vi "Initialise.vi"(8 "error in (no error)":errorcluster, 11 "JsonEvents in":refnum<class "JsonEvents.lvclass">) -> (0 "error out":errorcluster, 3 "JsonEvents out":refnum<class "JsonEvents.lvclass">)   [LabVIEW 2020, in "wamplv.lvlib" / "JsonEvents.lvclass"]
uses:
  JsonEvents.lvclass
  WAMP Client/Private/TypeDef/EVENT payload (JSON).ctl
  WAMP Client/API/TypeDefs/INVOCATION payload.ctl
  Invocation Request ID/Invocation Request ID.lvclass
  WAMP Client/API/TypeDefs/RESULT payload (JSON).ctl
  WAMP Client/API/TypeDefs/Error or abort detail (JSON).ctl
  JsonEvents.lvclass/JsonEvents.ctl
  EventsParent/Events.lvclass
  wamplv.lvlib
  WAMP Client/WAMP Client.lvclass
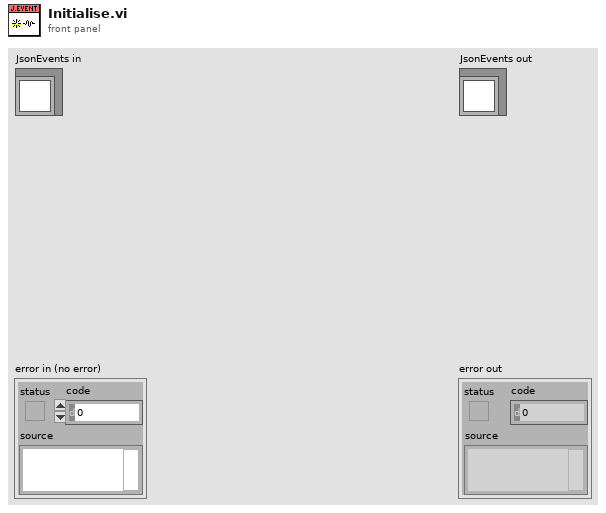
[diagram p1: front panel]
types:
  T1 = typedef "wamplv.lvlib/EVENT payload (JSON).ctl" = cluster{"Publication ID":u64, "Topic":string, "Arguments Payload":string, "ArgumentKw Payload":string, "Details":string}
  T2 = typedef "wamplv.lvlib/WAMP Client.lvclass/INVOCATION payload.ctl" = cluster{"Arguments":string, "ArgumentKw":string, "Procedure URI":string, "Details":string, "Registration ID":u64, "Invocation Request ID":refnum<class "Invocation Request ID.lvclass">}
  T3 = typedef "wamplv.lvlib/WAMP Client.lvclass/RESULT payload (JSON).ctl" = cluster{"Topic":string, "Arguments Payload":string, "ArgumentKw Payload":string, "Details":string, "Error/Abort details (JSON)":T4}
  T4 = typedef "wamplv.lvlib/Error or abort detail (JSON).ctl" = cluster{"Error URI":string, "Error Arguments":string, "Error ArgumentKw":string, "Error Details":string}
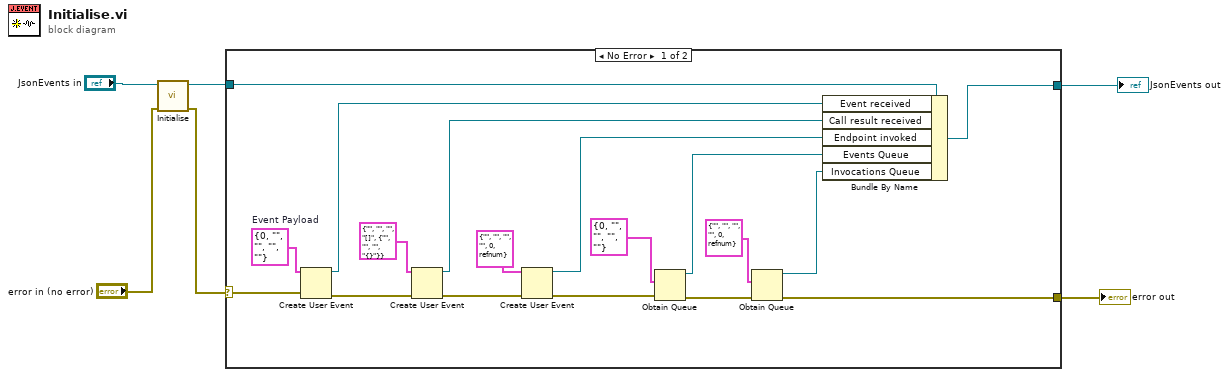
[diagram p0: block diagram]
diagram:
  n1 = call-parent "Initialise.vi"("error in (no error)"="error in (no error)", "EventsParent in"="JsonEvents in") -> ("error out"=w1:errorcluster, "EventsParent out"=w3:refnum<class "JsonEvents.lvclass">)  [unwired: 8 in]
  n2 = case shown="No Error" w1 {
    selector: w1 -> [w14 w25]
    tunnel: w3 -> [w24 w26]
    tunnel: [w23 w26] -> w6
    tunnel: [w7 w25] -> w5
    frame No Error {
      w22 = T1 {"Publication ID"=0, "Topic"="", "Arguments Payload"="", "ArgumentKw Payload"="", "Details"=""}  # Event Payload
      n3 = Create User Event(user event datatype=w22, error in=w14) -> (user event=w17:refnum<user-event>, error out=w20:errorcluster)
      n4 = Create User Event(user event datatype=T3 {"Topic"="", "Arguments Payload"="", "ArgumentKw Payload"="", "Details"="[]", "Error/Abort details (JSON)"={"Error URI"="", "Error Arguments"="", "Error ArgumentKw"="", "Error Details"="{}"}} ("RESULT Payload"), error in=w20) -> (user event=w16:refnum<user-event>, error out=w18:errorcluster)
      n5 = Create User Event(user event datatype=T2 {"Arguments"="", "ArgumentKw"="", "Procedure URI"="", "Details"="", "Registration ID"=0, "Invocation Request ID"=refnum} ("INVOCATION payload"), error in=w18) -> (user event=w15:refnum<user-event>, error out=w13:errorcluster)
      n6 = Obtain Queue(element data type=T1 {"Publication ID"=0, "Topic"="", "Arguments Payload"="", "ArgumentKw Payload"="", "Details"=""} ("Cluster"), error in (no error)=w13) -> (queue out=w9:refnum<queue>, error out=w12:errorcluster)  [unwired: 3 in, 1 out]
      n7 = Obtain Queue(element data type=T2 {"Arguments"="", "ArgumentKw"="", "Procedure URI"="", "Details"="", "Registration ID"=0, "Invocation Request ID"=refnum} ("INVOCATION payload"), error in (no error)=w12) -> (queue out=w8:refnum<queue>, error out=w7:errorcluster)  [unwired: 3 in, 1 out]
      n8 = Bundle By Name(cluster=w24, "Event received"=w17, "Call result received"=w16, "Endpoint invoked"=w15, "Events Queue"=w9, "Invocations Queue"=w8) -> (w23:refnum<class "JsonEvents.lvclass">)
    }
    frame Error {
    }
  }
  "error out" <- w5
  "JsonEvents out" <- w6
